vi "test init proc.vi"() -> ()   [LabVIEW 2013, in "CLFN tests.lvlib"]
uses:
  CLFN tests.lvlib
  <vilib>/NI/Tag Bus Module Framework/runtime/execution settings.ctl
  <vilib>/NI/Tag Bus/table/data table.ctl
  <vilib>/NI/Tag Bus/dictionary/full data dictionary.ctl
  <vilib>/NI/Tag Bus Module Framework/runtime/TBM module execution interface.lvclass
  <vilib>/NI/Tag Bus/dictionary/data dictionary.lvclass
  <vilib>/NI/Tag Bus/table/data table.lvlib
panel:
  in  "params/results default data":T1={"Double"=[2.0, 4.0, 6.0], "Single"=[3.0, 5.0, 7.0], "I64"=[], "I32"=[], "I16"=[], "I8"=[], "U64"=[], "U32"=[], "U16"=[], "U8"=[], "Boolean"=[], "String"=[], "Array of Double"=[], "Array of Single"=[], "Array of I64"=[], "Array of I32"=[], "Array of I16"=[], "Array of I8"=[], "Array of U64"=[], "Array of U32"=[], "Array of U16"=[], "Array of U8"=[], "Array of Boolean"=[], "Array of String"=[]}
  in  "resultdict":T2={"Double"=["result_dbl_1", "ghgr", "tnht"], "Single"=["asdadasd", "result_sgl_1", "sadbgh"], "I64"=[], "I32"=[], "I16"=[], "I8"=[], "U64"=[], "U32"=[], "U16"=[], "U8"=[], "Boolean"=[], "String"=[], "Array of Double"=[], "Array of Single"=[], "Array of I64"=[], "Array of I32"=[], "Array of I16"=[], "Array of I8"=[], "Array of U64"=[], "Array of U32"=[], "Array of U16"=[], "Array of U8"=[], "Array of Boolean"=[], "Array of String"=[]}
  in  "paramdict":T2={"Double"=["", "param_dbl_1", "someth"], "Single"=["asdasd", "asd", "param_sgl_1"], "I64"=[], "I32"=[], "I16"=[], "I8"=[], "U64"=[], "U32"=[], "U16"=[], "U8"=[], "Boolean"=[], "String"=[], "Array of Double"=[], "Array of Single"=[], "Array of I64"=[], "Array of I32"=[], "Array of I16"=[], "Array of I8"=[], "Array of U64"=[], "Array of U32"=[], "Array of U16"=[], "Array of U8"=[], "Array of Boolean"=[], "Array of String"=[]}
  in  "path":path=path "C:/Users/Daniel/Desktop/dlltesting/Windows/debug/platyplugin.dll"
  out "lvdataclusterout":T1={"Double"=[28.0, 4.0, 6.0], "Single"=[3.0, 11.0, 7.0], "I64"=[], "I32"=[], "I16"=[], "I8"=[], "U64"=[], "U32"=[], "U16"=[], "U8"=[], "Boolean"=[], "String"=[], "Array of Double"=[], "Array of Single"=[], "Array of I64"=[], "Array of I32"=[], "Array of I16"=[], "Array of I8"=[], "Array of U64"=[], "Array of U32"=[], "Array of U16"=[], "Array of U8"=[], "Array of Boolean"=[], "Array of String"=[]}
  out "execSettings":T3={"reads inputs"=FALSE, "processes data"=TRUE, "writes outputs"=FALSE}
  out "init return":i32
  out "procreturn":i32
  out "element":errorcluster
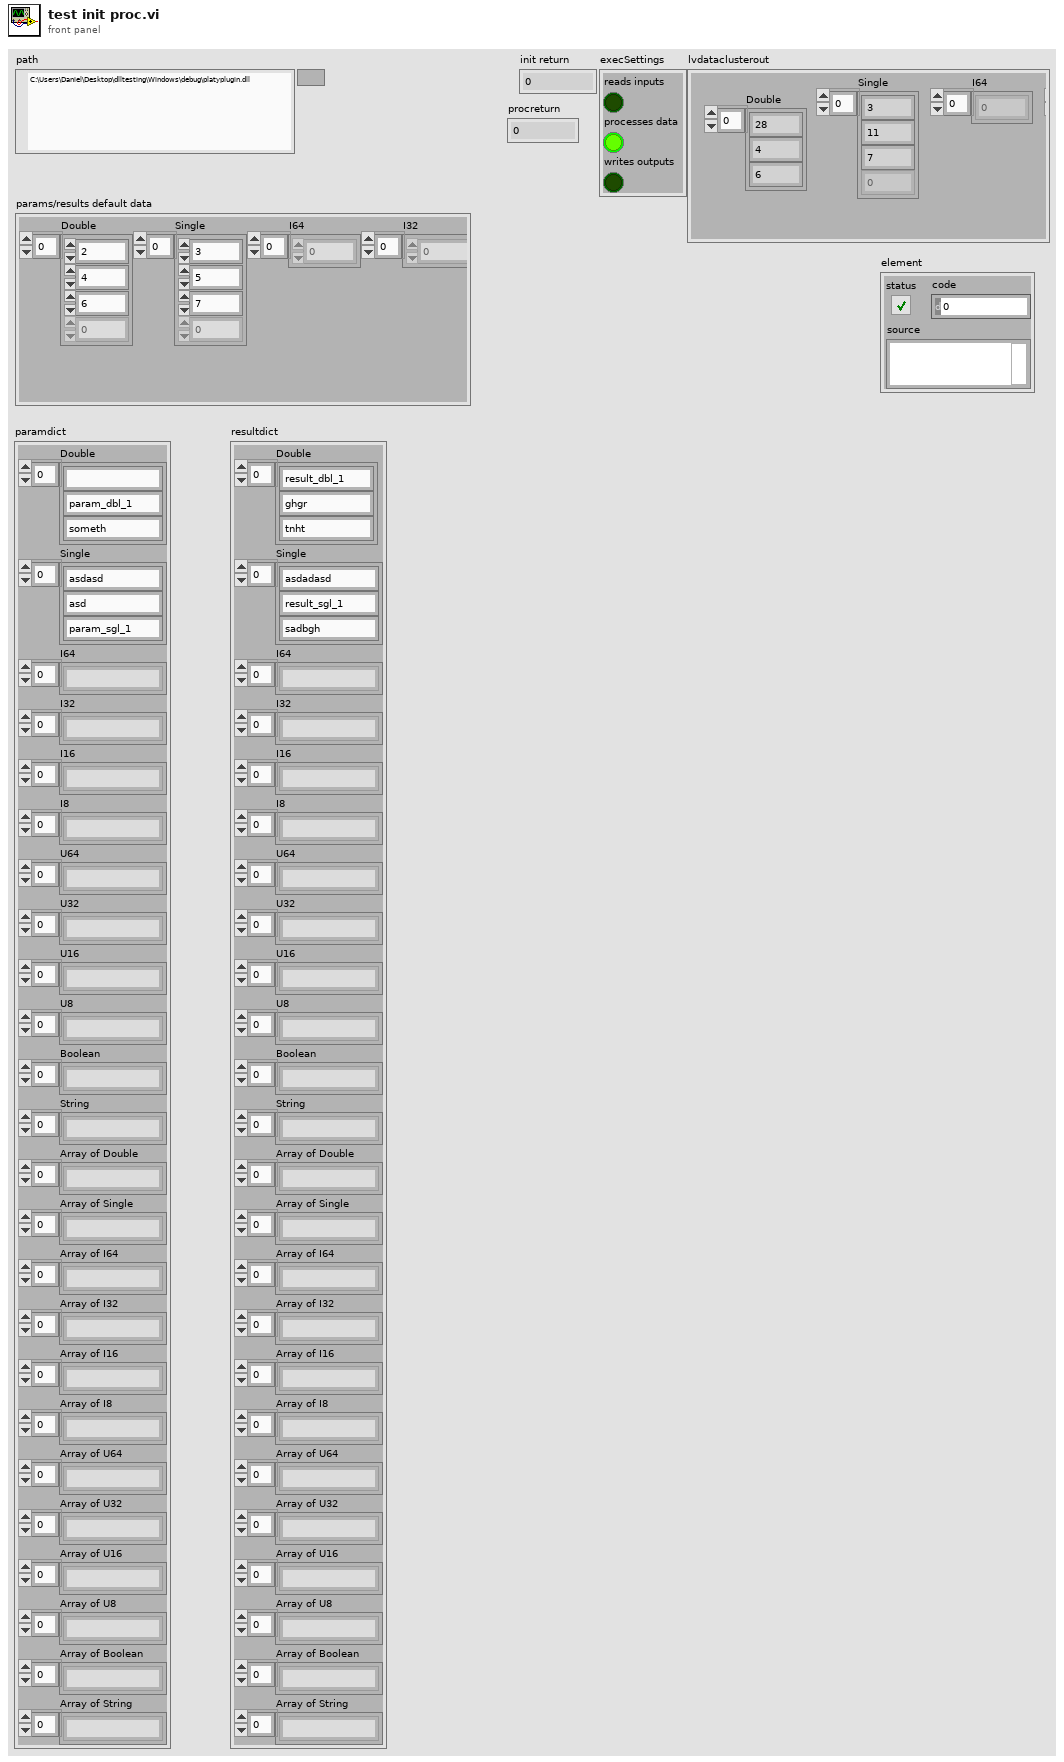
[diagram p1: front panel]
types:
  T1 = typedef "tag bus.lvlib/data table.lvlib/data table.ctl" = cluster{"Double":dbl[], "Single":sgl[], "I64":i64[], "I32":i32[], "I16":i16[], "I8":i8[], "U64":u64[], "U32":u32[], "U16":u16[], "U8":u8[], "Boolean":bool[], "String":string[], "Array of Double":cluster{"DBL Array":dbl[]}[], "Array of Single":cluster{"SGL Array":sgl[]}[], "Array of I64":cluster{"I64 Array":i64[]}[], "Array of I32":cluster{"I32 Array":i32[]}[], "Array of I16":cluster{"I16 Array":i16[]}[], "Array of I8":cluster{"I8 Array":i8[]}[], "Array of U64":cluster{"U64 Array":u64[]}[], "Array of U32":cluster{"U32 Array":u32[]}[], "Array of U16":cluster{"U16 Array":u16[]}[], "Array of U8":cluster{"U8 Array":u8[]}[], "Array of Boolean":cluster{"Boolean Array":bool[]}[], "Array of String":cluster{"String Array":string[]}[]}
  T2 = typedef "tag bus.lvlib/data dictionary.lvclass/full data dictionary.ctl" = cluster{"Double":string[], "Single":string[], "I64":string[], "I32":string[], "I16":string[], "I8":string[], "U64":string[], "U32":string[], "U16":string[], "U8":string[], "Boolean":string[], "String":string[], "Array of Double":string[], "Array of Single":string[], "Array of I64":string[], "Array of I32":string[], "Array of I16":string[], "Array of I8":string[], "Array of U64":string[], "Array of U32":string[], "Array of U16":string[], "Array of U8":string[], "Array of Boolean":string[], "Array of String":string[]}
  T3 = typedef "TBM module execution interface.lvclass/execution settings.ctl" = cluster{"reads inputs":bool, "processes data":bool, "writes outputs":bool}
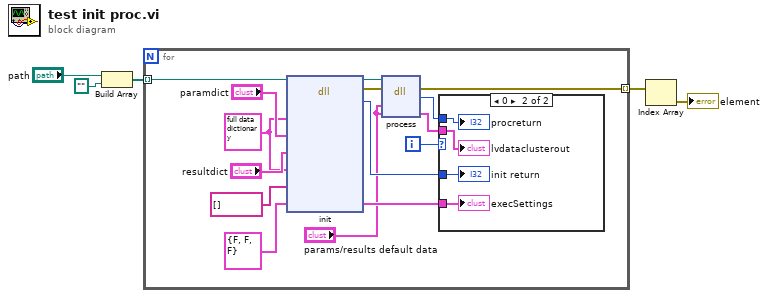
[diagram p0: block diagram]
diagram:
  n1 = Build Array("path", path "") -> (w3:path[])
  n2 = for {
    tunnel: w3 -> [w16] mode=indexing
    tunnel: [w20] -> w2 mode=indexing
    i -> [w19]
    w7 = T2 {"Double"=[], "Single"=[], "I64"=[], "I32"=[], "I16"=[], "I8"=[], "U64"=[], "U32"=[], "U16"=[], "U8"=[], "Boolean"=[], "String"=[], "Array of Double"=[], "Array of Single"=[], "Array of I64"=[], "Array of I32"=[], "Array of I16"=[], "Array of I8"=[], "Array of U64"=[], "Array of U32"=[], "Array of U16"=[], "Array of U8"=[], "Array of Boolean"=[], "Array of String"=[]} ("idict")
    n3 = dll-call lib="?" fn="init"(path in=w16, "idict"=w7, "pdict"="paramdict", "rdict"="resultdict", "odict"=w7, "args"=string[] [] ("I64"), "execSettings"=T3 {"reads inputs"=FALSE, "processes data"=FALSE, "writes outputs"=FALSE} ("execution settings")) -> (path out=w15:path, error out=w14:errorcluster, "return type"=w11:i32, "execSettings"=w13:T3)  [unwired: 7 in]
    n4 = dll-call lib="?" fn="process"(path in=w15, error in=w14, "lvdataclusterin"="params/results default data", "params/results default data") -> (error out=w20:errorcluster, "return type"=w18:i32, w17:T1)  [unwired: 2 in, 1 out]
    n5 = case shown="0" w19 {
      tunnel: w18 -> [_ w24]
      tunnel: w17 -> [_ w21]
      tunnel: w13 -> [_ w22]
      tunnel: w11 -> [_ w23]
      frame Default {
      }
      frame 0 {
        "procreturn" <- w24
        "init return" <- w23
        "execSettings" <- w22
        "lvdataclusterout" <- w21
      }
    }
  }
  n6 = Index Array(array=w2) -> (element=→"element":errorcluster)  [unwired: 1 in]
